vi "LoadClassesInheritanceTree.vi"(8 "error in (no error)":errorcluster, 9 "TreeControl":refnum<vi>, 10 "Project":refnum<vi>) -> (0 "error out":errorcluster, 1 "Classes":refnum<vi>[](array[refnum]), 2 "ClassesNames":string[](array[string]))   [LabVIEW 2014, in "ClassInheritanceEditor.lvlib" / "ClassInheritanceEditor.lvclass"]
uses:
  ClassInheritanceEditor.lvclass
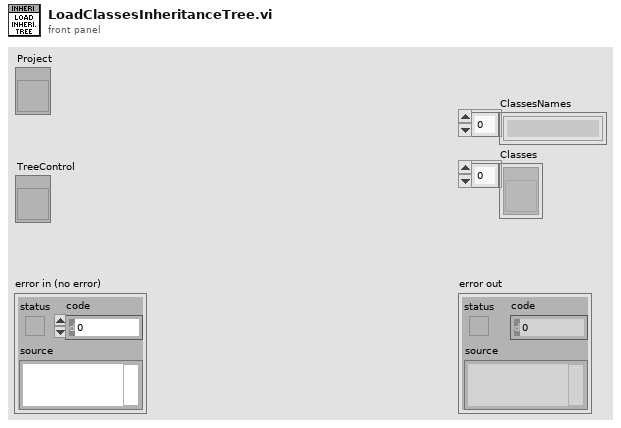
[diagram p1: front panel]
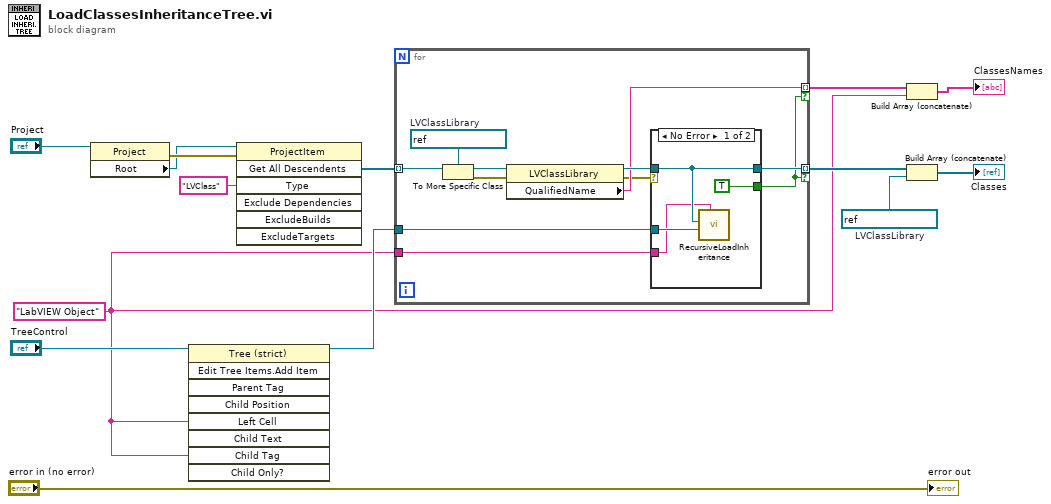
[diagram p0: block diagram]
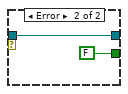
[diagram p2: hidden frame]
diagram:
  w3 = refnum<vi> refnum  # LVClassLibrary
  w1 = "LabVIEW Object" ("Parent Tag")
  n1 = property class="Project"(reference="Project") -> (error out=w11:errorcluster, "Root"=w10:refnum<vi>)  [unwired: 1 in, 1 out]
  n2 = invoke on="Invoke Node" class="Tree (strict)" method="Edit Tree Items.Add Item"(reference="TreeControl", "Left Cell"=w1, "Child Tag"=w1) -> (reference out=w5:refnum<vi>)  [unwired: 6 in, 8 out]
  n3 = invoke class="ProjectItem" method="Get All Descendents"(reference=w10, error in=w11, "Type"="LVClass") -> ("All Descendents"=w8:refnum<vi>[])  [unwired: 4 in, 6 out]
  n4 = for {
    tunnel: w8 -> [w22] mode=indexing
    tunnel: [w20] -> w9 mode=indexing if=w16
    tunnel: [w18] -> w7 mode=indexing if=w16
    tunnel: w5 -> [w23]
    tunnel: w1 -> [w15]
    w25 = refnum<vi> refnum  # LVClassLibrary
    n5 = To More Specific Class(target class=w25, reference=w22) -> (specific class reference=w24:refnum<vi>, error out=w19:errorcluster)  [unwired: 1 in]
    n6 = property class="LVClassLibrary"(reference=w24, error in=w19) -> (reference out=w21:refnum<vi>, error out=w17:errorcluster, "QualifiedName"=w20:string)
    n7 = case shown="No Error" w17 {
      tunnel: w23 -> [w29 _]
      tunnel: w21 -> [w28 w31]
      tunnel: [w28 w31] -> w18
      tunnel: [TRUE FALSE] -> w16
      tunnel: w15 -> [w26 _]
      frame No Error {
        n8 = call "RecursiveLoadInheritance.vi"("TopLevelParentTag"=w26, "TreeControl"=w29, "Class"=w28) -> ()  [unwired: 8 in, 1 out]
      }
      frame Error {
      }
    }
  }
  n9 = Build Array (concatenate)(w9, w1) -> (→"ClassesNames":string[])
  n10 = Build Array (concatenate)(w7, w3) -> (→"Classes":refnum<vi>[])
  "error out" <- "error in (no error)"
